vi "SendPropertyValues.vi"(6 "Value of Property":string, 7 "Property":string, 8 "error in (no error)":errorcluster, 9 "appKey":string, 10 "Beginning of Url":string, 11 "Refnum in":T1) -> (0 "error out":errorcluster, 1 "appKey out":string, 2 "url out":string, 3 "Refnum out":T1, 5 "body":string)   [LabVIEW 2015]
uses:
  <vilib>/httpClient/ClientHandle.ctl
  <vilib>/httpClient/PUTBuffer.vi
  <vilib>/httpClient/LabVIEWHTTPClient.lvlib
panel:
  out "Final url":string
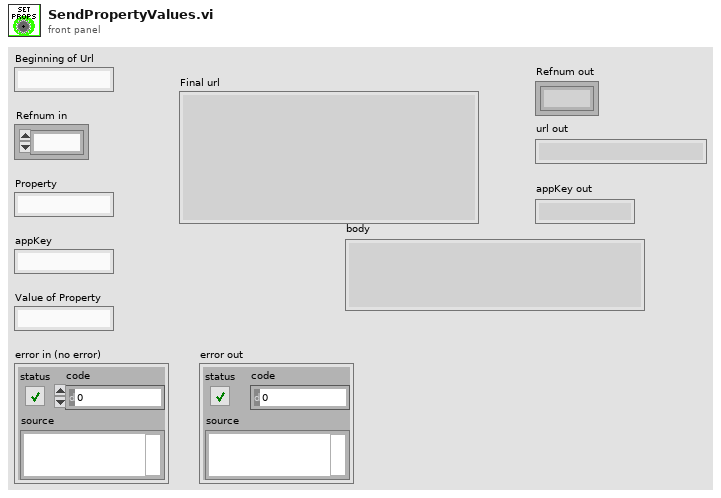
[diagram p1: front panel]
types:
  T1 = typedef "LabVIEWHTTPClient.lvlib/ClientHandle.ctl" = refnum<k1>
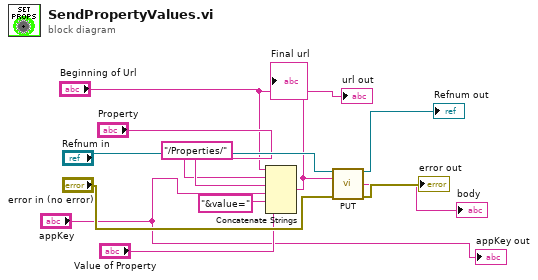
[diagram p0: block diagram]
diagram:
  n1 = Concatenate Strings("Beginning of Url", "/Properties/" ("string"), "Property", "appKey", "&value=" ("string"), "Value of Property") -> (w8:string)
  "Final url" <- w8
  n2 = call-poly <vilib>:"PUT.vi"("client handle"="Refnum in", "url"=w8, "error in (no error)"="error in (no error)") -> ("client handle out"=→"Refnum out":T1, "body"=→"body":string, "error out"=→"error out":errorcluster)  [unwired: 9 in, 1 out]
  "url out" <- "Beginning of Url"
  "appKey out" <- "appKey"
